vi "write_key_integer.vi"(7 "table":string="nipm", 8 "error in (no error)":errorcluster, 9 "value":i64, 10 "key":string="version", 11 "toml in":refnum<class "toml.lvclass">) -> (0 "error out":errorcluster, 3 "toml out":refnum<class "toml.lvclass">)   [LabVIEW 2020, in "toml.lvclass"]
uses:
  toml.lvclass
  toml.lvclass/toml.ctl
  Doc/Doc.lvclass
  Table/Table.lvclass
  Item/Item.lvclass
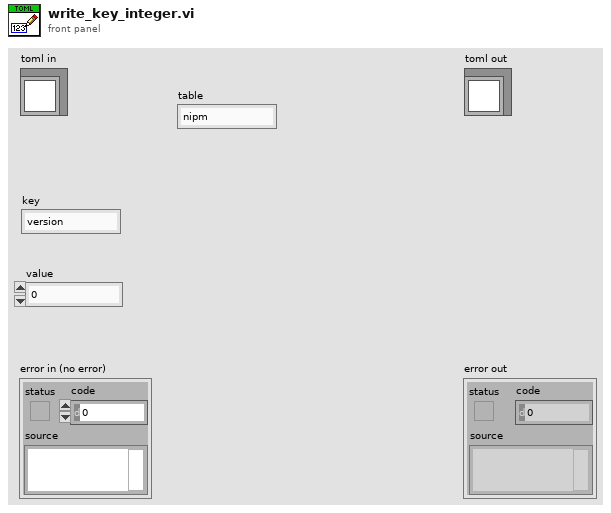
[diagram p1: front panel]
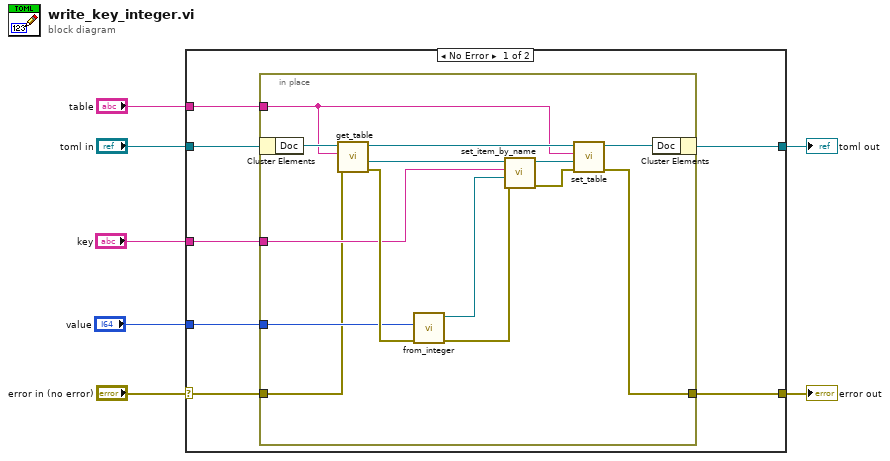
[diagram p0: block diagram]
diagram:
  n1 = case shown="No Error" "error in (no error)" {
    selector: "error in (no error)" -> [w8 w30]
    tunnel: [w9 w30] -> w6
    tunnel: [w13 w29] -> w4
    tunnel: "toml in" -> [w14 w29]
    tunnel: "table" -> [w12 _]
    tunnel: "key" -> [w11 _]
    tunnel: "value" -> [w10 _]
    frame No Error {
      n2 = in-place {
        in-place-border: w12 -> [w20]
        in-place-border: w11 -> [w19]
        in-place-border: w10 -> [w18]
        in-place-border: [w16] -> w9
        in-place-border: w8 -> [w15]
        n3 = in-place-cluster #1(w14) -> ("Doc"=w22:refnum<class "Doc.lvclass">)
        n4 = call "get_table.vi"("error in (no error)"=w15, "table_name"=w20, "Doc in"=w22) -> ("error out"=w27:errorcluster, "Table"=w26:refnum<class "Table.lvclass">, "Doc out"=w24:refnum<class "Doc.lvclass">)  [unwired: 6 in]
        n5 = call "from_integer.vi"("error in (no error)"=w27, "value"=w18) -> ("error out"=w28:errorcluster, "Item out"=w25:refnum<class "Item.lvclass">)  [unwired: 8 in]
        n6 = call "set_item_by_name.vi"("error in (no error)"=w28, "Item"=w25, "item_name"=w19, "Table in"=w26) -> ("error out"=w17:errorcluster, "Table out"=w23:refnum<class "Table.lvclass">)  [unwired: 6 in]
        n7 = call "set_table.vi"("error in (no error)"=w17, "Table"=w23, "table_name"=w20, "Doc in"=w24) -> ("error out"=w16:errorcluster, "Doc out"=w21:refnum<class "Doc.lvclass">)  [unwired: 6 in]
        n8 = in-place-cluster #1("Doc"=w21) -> (w13:refnum<class "toml.lvclass">)
      }
    }
    frame Error {
    }
  }
  "error out" <- w6
  "toml out" <- w4
